vi "Get Thread Configuration.vi"(8 "error in (no error)":errorcluster, 11 "Component Configuration in":refnum<class "GE Reflective Memory Configurations.lvclass">) -> (0 "error out":errorcluster, 2 "Thread Configuration":refnum<class "Configuration.lvclass">, 3 "Component Configuration out":refnum<class "GE Reflective Memory Configurations.lvclass">)   [LabVIEW 2020, in "GE Reflective Memory.lvlib" / "GE Reflective Memory Configurations.lvclass"]
uses:
  GE Reflective Memory Configurations.lvclass
  DSF Core.lvlibp/Classes/Configuration/Configuration.lvclass
  Thread/Thread Configuration.lvclass
  C:/Users/nitest/Desktop/Git 2020/niveristand-data-sharing-framework-custom-device-plugins/Components/DSF Core.lvlibp/Classes/Configuration/Configuration.lvclass
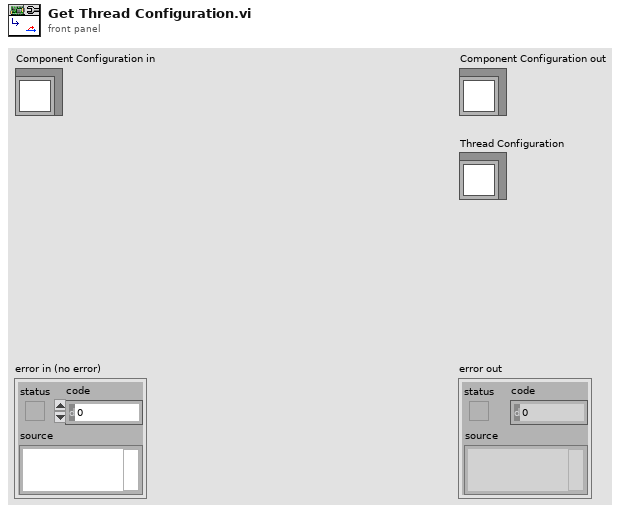
[diagram p1: front panel]
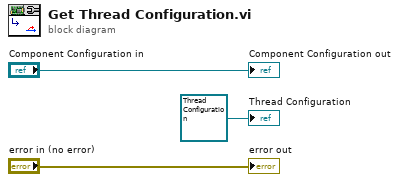
[diagram p0: block diagram]
diagram:
  "error out" <- "error in (no error)"
  "Component Configuration out" <- "Component Configuration in"
  "Thread Configuration" <- refnum<class "Thread Configuration.lvclass"> refnum ("GE Reflective Memory.lvlib:Thread Configuration.lvclass")
